vi "cw_2_5.vi"() -> ()   [LabVIEW 2022 SP3]
panel:
  in  "stop":bool
  in  "loop delay [ms]":u32=10
  out "Waveform Chart":i16(graph)
  in  "duty cycle [%]":i32=75
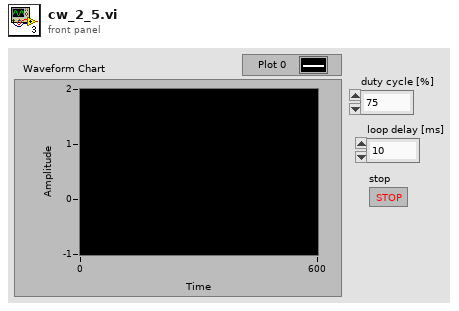
[diagram p1: front panel]
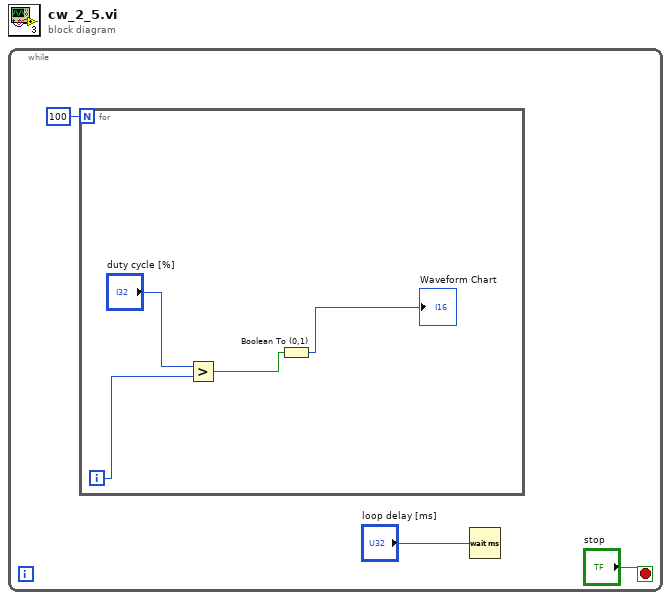
[diagram p0: block diagram]
diagram:
  n1 = while {
    stop <- "stop" stop-if-true
    n2 = for {
      N: 100 -> [_]
      i -> [w7]
      n3 = Greater?(x="duty cycle [%]", y=w7) -> (0:w5:bool)
      n4 = Boolean To (0,1)(Boolean=w5) -> (0, 1=→"Waveform Chart":i16)
    }
    n5 = Wait (ms)(milliseconds to wait="loop delay [ms]") -> ()  [unwired: 1 out]
  }
